vi "GraphAndChartNotesMarcoGonzalez.vi"() -> ()   [LabVIEW 2012]
panel:
  out "Waveform Chart":dbl[](graph)
  out "Waveform Graph":dbl[][](graph)
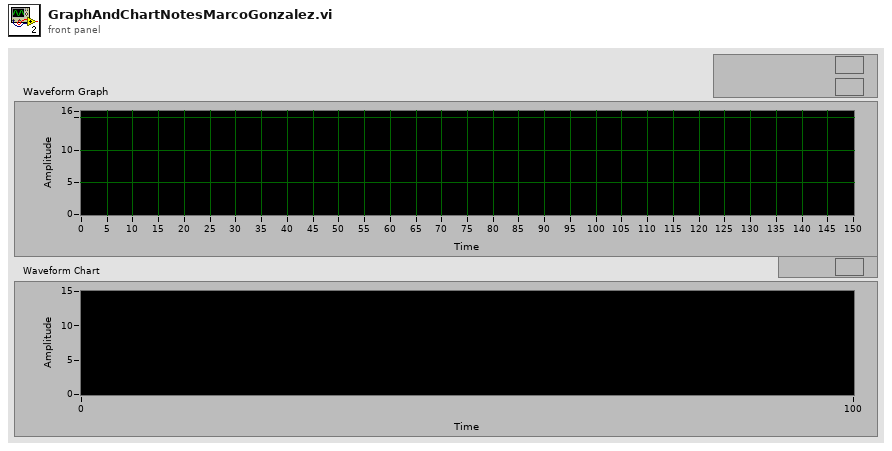
[diagram p1: front panel]
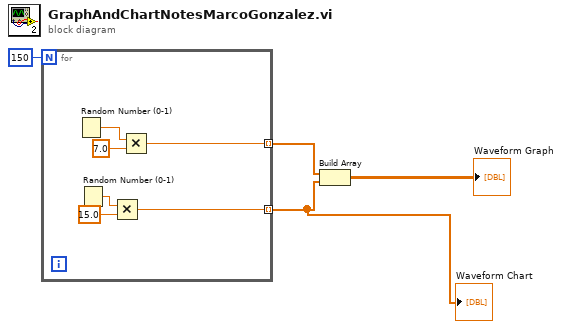
[diagram p0: block diagram]
diagram:
  n1 = for {
    N: 150 -> [_]
    tunnel: [w5] -> w3 mode=indexing
    tunnel: [w6] -> w1 mode=indexing
    n2 = Random Number (0-1)() -> (number: 0 to 1=w9:dbl)
    n3 = Random Number (0-1)() -> (number: 0 to 1=w8:dbl)
    n4 = Multiply(x=w8, y=15.0) -> (x*y=w6:dbl)
    n5 = Multiply(x=w9, y=7.0) -> (x*y=w5:dbl)
  }
  "Waveform Chart" <- w1
  n6 = Build Array(w3, w1) -> (→"Waveform Graph":dbl[][])
